vi "get_number_of_images.vi"(8 "error in (no error)":errorcluster, 11 "ImageCollection in":refnum<class "ImageCollection.lvclass">) -> (0 "error out":errorcluster, 2 "size":i32, 3 "ImageCollection out":refnum<class "ImageCollection.lvclass">)   [LabVIEW 2010, in "ImageCollection.lvclass"]
uses:
  ImageCollection.lvclass
  ImageCollection.lvclass/ImageCollection.ctl
  libraries/TIFFManagement/TIFFManagement.lvlib
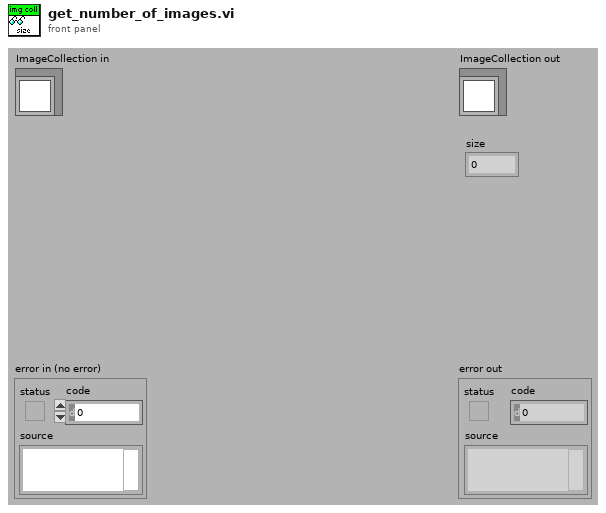
[diagram p1: front panel]
types:
  T1 = typedef "ImageCollection.lvclass/storage_mode_enum.ctl" = enum16{"RAM", "single files", "multipage TIFF (read-only)"}
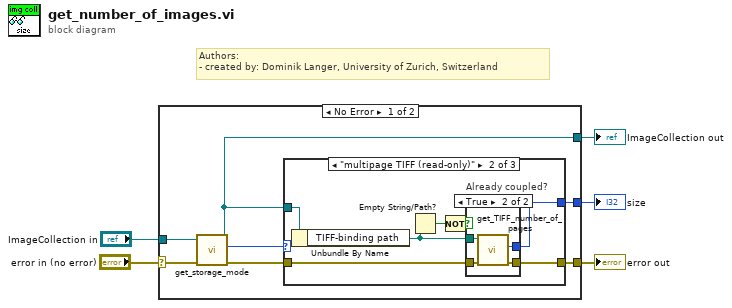
[diagram p0: block diagram]
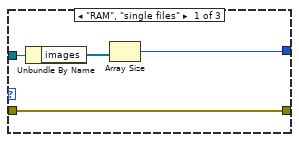
[diagram p2: hidden frame]
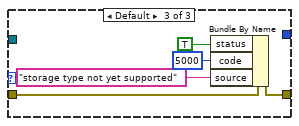
[diagram p4: hidden frame]
diagram:
  # "Authors: \n- created by: Dominik Langer, University of Zurich, Switzerland"
  n1 = case shown="No Error" "error in (no error)" {
    selector: "error in (no error)" -> [w11 w35]
    tunnel: [w12 w35] -> w4
    tunnel: [w7 w34] -> w2
    tunnel: "ImageCollection in" -> [w9 w34]
    tunnel: [w6 _] -> w1
    frame No Error {
      n2 = call-dynamic "get_storage_mode.vi"("error in (no error)"=w11, "ImageCollection.lvclass in"=w9) -> ("error out"=w10:errorcluster, "storage type"=w8:T1, "ImageCollection.lvclass out"=w7:refnum<class "ImageCollection.lvclass">)  [unwired: 7 out]
      n3 = case shown="\"multipage TIFF (read-only)\"" w8 {
        tunnel: w10 -> [w15 w22 w33]
        tunnel: w7 -> [w16 w23 _]
        tunnel: [w15 w21 w32] -> w12
        tunnel: [w13 w20 _] -> w6
        frame "RAM", "single files" {
          n4 = Unbundle By Name(w16) -> ("images"=w14:refnum<class "Image.lvclass">[])
          n5 = Array Size(array=w14) -> (size(s)=w13:i32)
        }
        frame "multipage TIFF (read-only)" {
          n6 = Unbundle By Name(w23) -> ("TIFF-binding path"=w19:path)
          n7 = Empty String/Path?(string/path=w19) -> (empty?=w18:bool)
          n8 = Not(x=w18) -> (.not. x?=w17:bool)
          n9 = case "Already coupled?" shown="True" w17 {
            tunnel: w22 -> [w24 w28]
            tunnel: [w24 w27] -> w21
            tunnel: [_ w26] -> w20
            tunnel: w19 -> [_ w25]
            frame False {
            }
            frame True {
              n10 = call "get_TIFF_number_of_pages.vi"("error in (no error)"=w28, "path in"=w25) -> ("error out"=w27:errorcluster, "number of pages"=w26:i32)  [unwired: 7 in, 1 out]
            }
          }
        }
        frame Default {
          n11 = Bundle By Name(cluster=w33, "status"=TRUE, "code"=5000, "source"="storage type not yet supported") -> (w32:errorcluster)
        }
      }
    }
    frame Error {
    }
  }
  "error out" <- w4
  "ImageCollection out" <- w2
  "size" <- w1
